vi "sug_query-select.vi"(7 "query type":T1) -> ()   [LabVIEW 2019]
uses:
  query type.ctl
  Durability/common/Global 1.vi
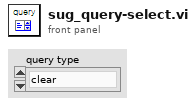
[diagram p1: front panel]
types:
  T1 = typedef "query type.ctl" = enum16{"clear", "capacitor set", "capacitor get"}
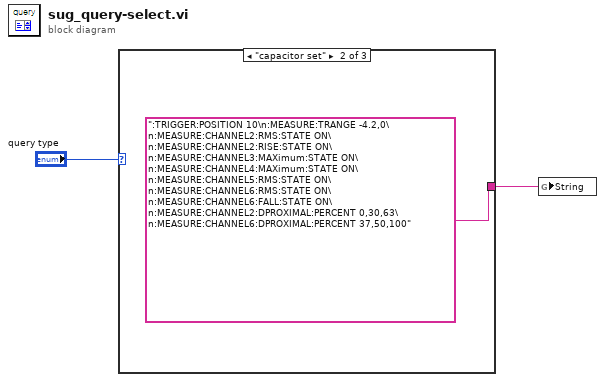
[diagram p0: block diagram]
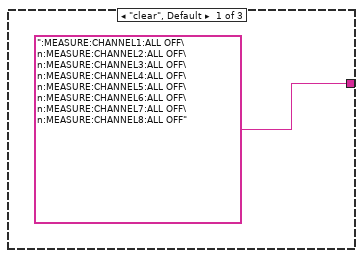
[diagram p2: hidden frame]
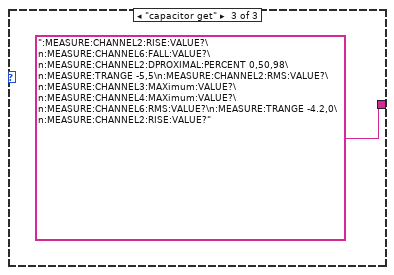
[diagram p3: hidden frame]
diagram:
  n1 = case shown="\"capacitor set\"" "query type" {
    tunnel: [":MEASURE:CHANNEL1:ALL OFF\n:MEASURE:CHANNEL2:ALL OFF\n:MEASURE:CHANNEL3:ALL OFF\n:MEASURE:CHANNEL4:ALL OFF\n:MEASURE:CHANNEL5:ALL OFF\n:MEASURE:CHANNEL6:ALL OFF\n:MEASURE:CHANNEL7:ALL OFF\n:MEASURE:CHANNEL8:ALL OFF" ":TRIGGER:POSITION 10\n:MEASURE:TRANGE -4.2,0\n:MEASURE:CHANNEL2:RMS:STATE ON\n:MEASURE:CHANNEL2:RISE:STATE ON\n:MEASURE:CHANNEL3:MAXimum:STATE ON\n:MEASURE:CHANNEL4:MAXimum:STATE ON\n:MEASURE:CHANNEL5:RMS:STATE ON\n:MEASURE:CHANNEL6:RMS:STATE ON\n:MEASURE:CHANNEL6:FALL:STATE ON\n:MEASURE:CHANNEL2:DPROXIMAL:PERCENT 0,30,63\n:MEASURE:CHANNEL6:DPROXIMAL:PERCENT 37,50,100" ":MEASURE:CHANNEL2:RISE:VALUE?\n:MEASURE:CHANNEL6:FALL:VALUE?\n:MEASURE:CHANNEL2:DPROXIMAL:PERCENT 0,50,98\n:MEASURE:TRANGE -5,5\n:MEASURE:CHANNEL2:RMS:VALUE?\n:MEASURE:CHANNEL3:MAXimum:VALUE?\n:MEASURE:CHANNEL4:MAXimum:VALUE?\n:MEASURE:CHANNEL6:RMS:VALUE?\n:MEASURE:TRANGE -4.2,0\n:MEASURE:CHANNEL2:RISE:VALUE?"] -> w1
    frame "clear", Default {
    }
    frame "capacitor set" {
    }
    frame "capacitor get" {
    }
  }
  n2 = global write "Global 1.vi" "String"(w1) -> ()
